vi "utility.TestItemTime.vi"(7 "TestTime_IN":T1, 8 "结束时间":timestamp, 9 "开始时间":timestamp, 10 "名称":string, 11 "序号":u64) -> (3 "TestTime_OUT":T1)   [LabVIEW 2012, in "Lib_UEL.ATE.lvlib" / "Lib_App.lvlib"]
uses:
  Lib_App.lvlib
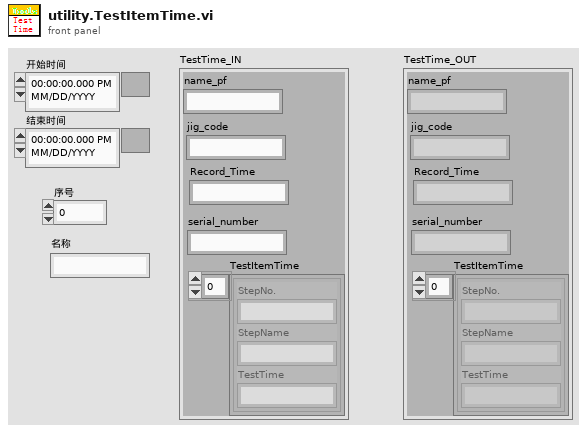
[diagram p1: front panel]
types:
  T1 = cluster{"name_pf":string, "jig_code":string, "Record_Time":string, "serial_number":string, "TestItemTime":cluster{"StepNo.":string, "StepName":string, "TestTime":string}[]}
  T2 = cluster{"StepNo.":string, "StepName":string, "TestTime":string}[]
  T3 = cluster{"StepNo.":string, "StepName":string, "TestTime":string}
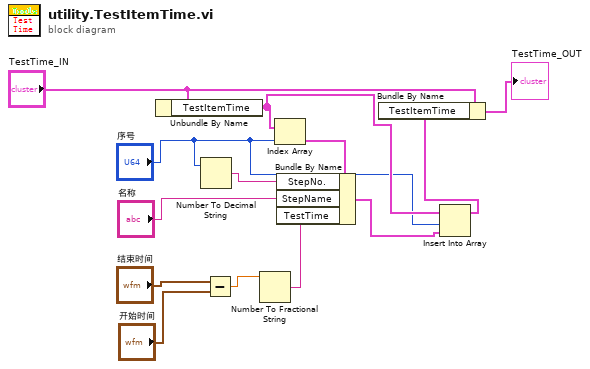
[diagram p0: block diagram]
diagram:
  n1 = Unbundle By Name("TestTime_IN") -> ("TestItemTime"=w5:T2)
  n2 = Number To Decimal String(number="序号") -> (decimal integer string=w12:string)  [unwired: 1 in]
  n3 = Subtract(x="结束时间", y="开始时间") -> (x-y=w8:dbl)
  n4 = Number To Fractional String(number=w8) -> (F-format string=w7:string)  [unwired: 3 in]
  n5 = Index Array(array=w5, index="序号") -> (element=w6:T3)
  n6 = Bundle By Name(cluster=w6, "StepNo."=w12, "StepName"="名称", "TestTime"=w7) -> (w3:T3)
  n7 = Insert Into Array(array=w5, index="序号", new element=w3) -> (w2:T2)
  n8 = Bundle By Name(cluster="TestTime_IN", "TestItemTime"=w2) -> (→"TestTime_OUT":T1)
